vi "SavePoints.vi"(10 "Data in":string[][](array[string]), 11 "XML File Path":path) -> (2 "Point":T1[](array[typedef]))   [LabVIEW 2017]
uses:
  Ctrls/Point.ctl
  <vilib>/Utility/xml.llb/Write to XML File(string).vi
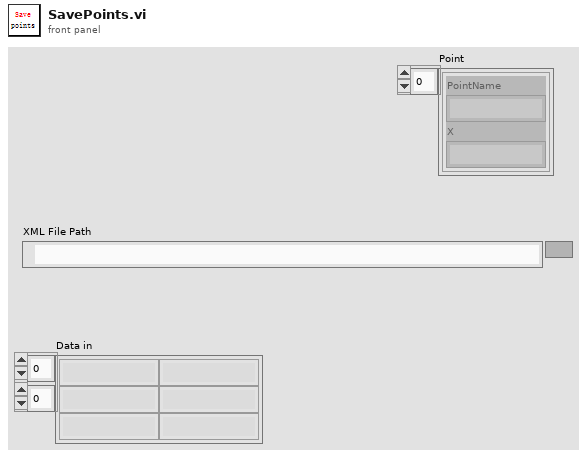
[diagram p1: front panel]
types:
  T1 = typedef "Point.ctl" = cluster{"PointName":string, "X":string}
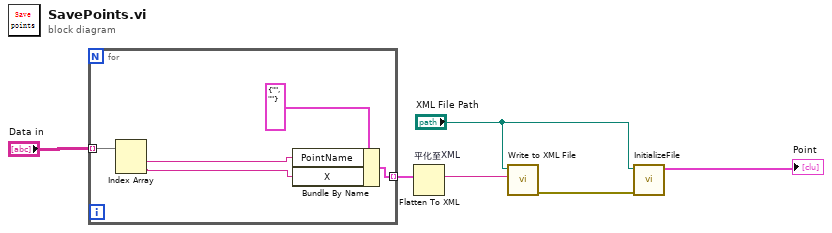
[diagram p0: block diagram]
diagram:
  n1 = for {
    tunnel: "Data in" -> [w11] mode=indexing
    tunnel: [w9] -> w2 mode=indexing
    n2 = Index Array(array=w11) -> (element #1=w10:string, element #2=w8:string)  [unwired: 2 in]
    n3 = Bundle By Name(cluster=T1 {"PointName"="", "X"=""}, "PointName"=w10, "X"=w8) -> (w9:T1)
  }
  n4 = Flatten To XML "平化至XML"(anything=w2) -> (xml string=w5:string)
  n5 = call-poly <vilib>:"Write to XML File.vi"("XML Input"=w5, "XML File Path"="XML File Path") -> ("error out"=w3:errorcluster)  [unwired: 7 in, 2 out]
  n6 = call "InitializeFile.vi"("error in (no error)"=w3, "XML File Path"="XML File Path") -> ("Point"=→"Point":T1[])  [unwired: 8 in, 1 out]
